vi "prompt - file save.vi"(11 "Path":path) -> (3 "message":string="PayloadID field cannot \nbe empty. Frame was\nnot added.")   [LabVIEW 2020, in "FrameEditor.lvlib"]
uses:
  FrameEditor.lvlib
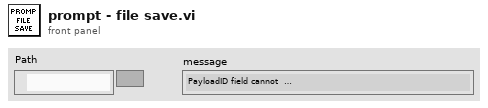
[diagram p1: front panel]
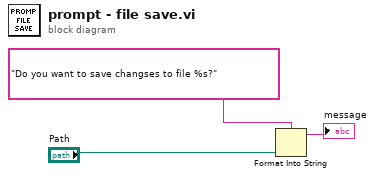
[diagram p0: block diagram]
diagram:
  n1 = Format Into String(format string="Do you want to save changses to file %s?" ("message"), "Path") -> (resulting string=→"message":string)  [unwired: 2 in, 1 out]
